vi "Rotate.vi"(8 "error in":errorcluster, 9 "speed(deg/s)":dbl=2.0 min=0.0, 10 "distance(deg)":dbl, 11 "Gantry in":refnum<class "Gantry.lvclass">) -> (0 "error out":errorcluster, 3 "Gantry out":refnum<class "Gantry.lvclass">)   [LabVIEW 2026, in "Gantry.lvclass"]
uses:
  Gantry.lvclass
  <instrlib>/Aerotech Automation1/Commands/Motion/typedefs/MoveIncremental parameters.ctl
  FlexWorktable/FlexWorktable.lvclass
  <instrlib>/Aerotech Automation1/Aerotech Automation1.lvlib
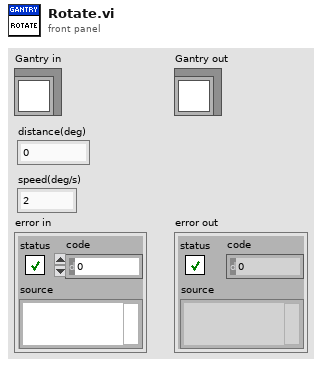
[diagram p1: front panel]
types:
  T1 = typedef "Aerotech Automation1.lvlib/MoveIncremental parameters.ctl" = cluster{"speeds":dbl[], "distances":dbl[], "axes":string[]}
  T2 = typedef "Virtual Modes.ctl" = enum16{"Nonvirtual", "Virtual"}
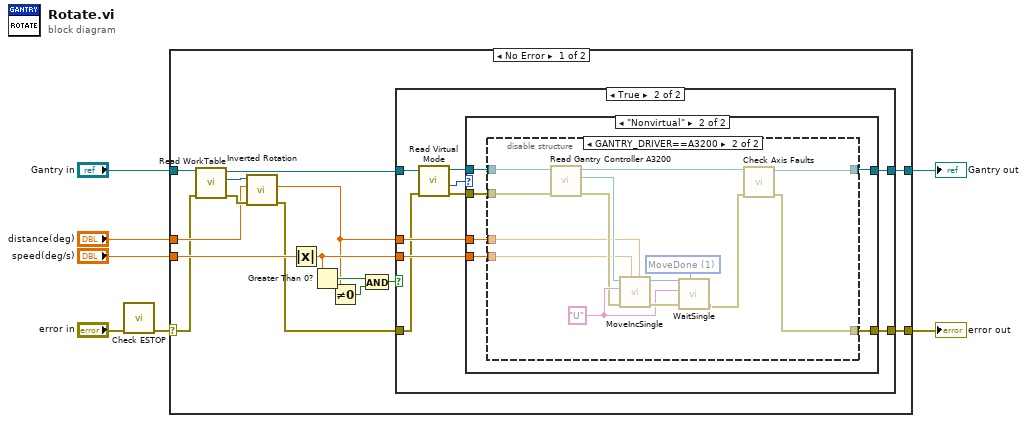
[diagram p0: block diagram]
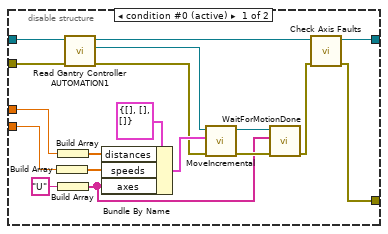
[diagram p4: hidden frame]
diagram:
  n1 = call "Check ESTOP.vi"("error in"="error in") -> ("error out"=w4:errorcluster)  [unwired: 10 in]
  n2 = case shown="No Error" w4 {
    selector: w4 -> [w9 w75]
    tunnel: [w22 w75] -> w7
    tunnel: [w16 w74] -> w6
    tunnel: "Gantry in" -> [w13 w74]
    tunnel: "distance(deg)" -> [w11 _]
    tunnel: "speed(deg/s)" -> [w21 _]
    frame No Error {
      n3 = call-dynamic "Read WorkTable.vi"("error in"=w9, "Gantry Class in"=w13) -> ("error out"=w14:errorcluster, "Worktable"=w15:refnum<class "FlexWorktable.lvclass">, "Gantry Class out"=w12:refnum<class "Gantry.lvclass">)  [unwired: 7 in]
      n4 = call "Inverted Rotation.vi"("error in (no error)"=w14, "Rotation in"=w11, "FlexWorktable in"=w15) -> ("error out"=w8:errorcluster, "Rotation out"=w10:dbl)  [unwired: 6 in, 1 out]
      n5 = Absolute Value(x=w21) -> (abs(x)=w20:dbl)
      n6 = Greater Than 0?(x=w20) -> (x > 0?=w18:bool)
      n7 = Not Equal To 0?(x=w10) -> (x != 0?=w17:bool)
      n8 = And(x=w18, y=w17) -> (x .and. y?=w19:bool)
      n9 = case shown="True" w19 {
        tunnel: w12 -> [w24 w29]
        tunnel: w8 -> [w23 w27]
        tunnel: [w23 w33] -> w22
        tunnel: w10 -> [_ w32]
        tunnel: w20 -> [_ w31]
        tunnel: [w24 w30] -> w16
        frame False {
        }
        frame True {
          n10 = call-dynamic "Read Virtual Mode.vi"("error in (no error)"=w27, "Gantry in"=w29) -> ("error out"=w26:errorcluster, "Virtual Mode"=w25:T2, "Gantry out"=w28:refnum<class "Gantry.lvclass">)  [unwired: 6 in, 1 out]
          n11 = case shown="\"Nonvirtual\"" w25 {
            tunnel: w26 -> [w34 w40]
            tunnel: [w34 w36] -> w33
            tunnel: w32 -> [_ w38]
            tunnel: w31 -> [_ w37]
            tunnel: [w35 w39] -> w30
            tunnel: w28 -> [w35 w41]
            frame "Virtual" {
            }
            frame "Nonvirtual" {
              n12 = disable-structure shown="GANTRY_DRIVER==A3200" {
                disable-tunnel: w41 -> [w59 w63]
                disable-tunnel: w40 -> [w58 w62]
                disable-tunnel: [w56 w60] -> w39
                disable-tunnel: w38 -> [w54 w65]
                disable-tunnel: w37 -> [w53 w64]
                disable-tunnel: [w42 w61] -> w36
                frame condition #0 (active) {
                  n13 = Build Array(w53) -> (w51:dbl[])
                  n14 = Build Array(w54) -> (w50:dbl[])
                  n15 = Build Array("U") -> (w45:string[])
                  n16 = call "Read Gantry Controller AUTOMATION1.vi"("error in (no error)"=w58, "Gantry in"=w59) -> ("error out"=w48:errorcluster, "Controller AUTOMATION1"=w47:refnum<k24>, "Gantry out"=w57:refnum<class "Gantry.lvclass">)  [unwired: 7 in]
                  n17 = Bundle By Name(cluster=T1 {"speeds"=[], "distances"=[], "axes"=[]} ("MoveIncremental parameters"), "distances"=w50, "speeds"=w51, "axes"=w45) -> (w49:T1)
                  n18 = call <instrlib>:"MoveIncremental.vi"("error in (no error)"=w48, "MoveIncremental parameters"=w49, "Controller Refnum"=w47) -> ("error out"=w46:errorcluster, "Controller Refnum out"=w44:refnum<k24>)  [unwired: 7 in]
                  n19 = call <instrlib>:"WaitForMotionDone.vi"("error in (no error)"=w46, "axes"=w45, "Controller Refnum"=w44) -> ("error out"=w43:errorcluster)  [unwired: 7 in, 1 out]
                  n20 = call "Check Axis Faults.vi"("error in (no error)"=w43, "Gantry in"=w57) -> ("error out"=w42:errorcluster, "Gantry out"=w56:refnum<class "Gantry.lvclass">)  [unwired: 8 in]
                }
                frame condition #1 {
                  w72 = 1 items=["InPosition", "MoveDone"] ("wait option?")
                  w70 = "U" ("axis name")
                  n21 = call "Read Gantry Controller A3200.vi"("error in (no error)"=w62, "Gantry in"=w63) -> ("error out"=w67:errorcluster, "A3200 controller out"=w66:refnum<k24>, "Gantry out"=w68:refnum<class "Gantry.lvclass">)  [unwired: 7 in]
                  n22 = call "MoveIncSingle.vi"("distance"=w65, "speed"=w64, "error in (no error)"=w67, "axis name"=w70, "controller in"=w66) -> ("error out"=w71:errorcluster, "controller out"=w73:refnum<k24>)  [unwired: 5 in]
                  n23 = call "WaitSingle.vi"("wait option?"=w72, "error in (no error)"=w71, "axis name"=w70, "controller in"=w73) -> ("error out"=w69:errorcluster)  [unwired: 5 in, 2 out]
                  n24 = call "Check Axis Faults.vi"("error in (no error)"=w69, "Gantry in"=w68) -> ("error out"=w61:errorcluster, "Gantry out"=w60:refnum<class "Gantry.lvclass">)  [unwired: 8 in]
                }
              }
            }
          }
        }
      }
    }
    frame Error {
    }
  }
  "error out" <- w7
  "Gantry out" <- w6
